vi "UI.vi"() -> ()   [LabVIEW 2017]
uses:
  <vilib>/vision/NI_Vision_Development_Module.lvlib
panel:
  out "Left side points":dbl[][](array[numeric])
  out "Bottom side points":dbl[][](array[numeric])
  out "Right side points":dbl[][](array[numeric])
  out "Top side points":dbl[][](array[numeric])
  out "time image processing":u32
  out "time load image":u32
  out "main Y":dbl[](array[numeric])
  out "main X":dbl[](array[numeric])
  out "corner":dbl[][](array[numeric])
  out "Y Resolution":i32
  out "X Resolution":i32
  out "testing 2":T1(plugin-control)
  out "black image":T1(plugin-control)
  out "buffer image":T1(plugin-control)
  in  "Path":path
  in  "Canny Parameters":T2={"Sigma"=1.0, "HThresh"=0.7, "LThres"=0.2, "WindowSize"=9}
  in  "Range (Threshold)":cluster{"Lower value":sgl, "Upper value":sgl}={"Lower value"=73.0, "Upper value"=255.0}
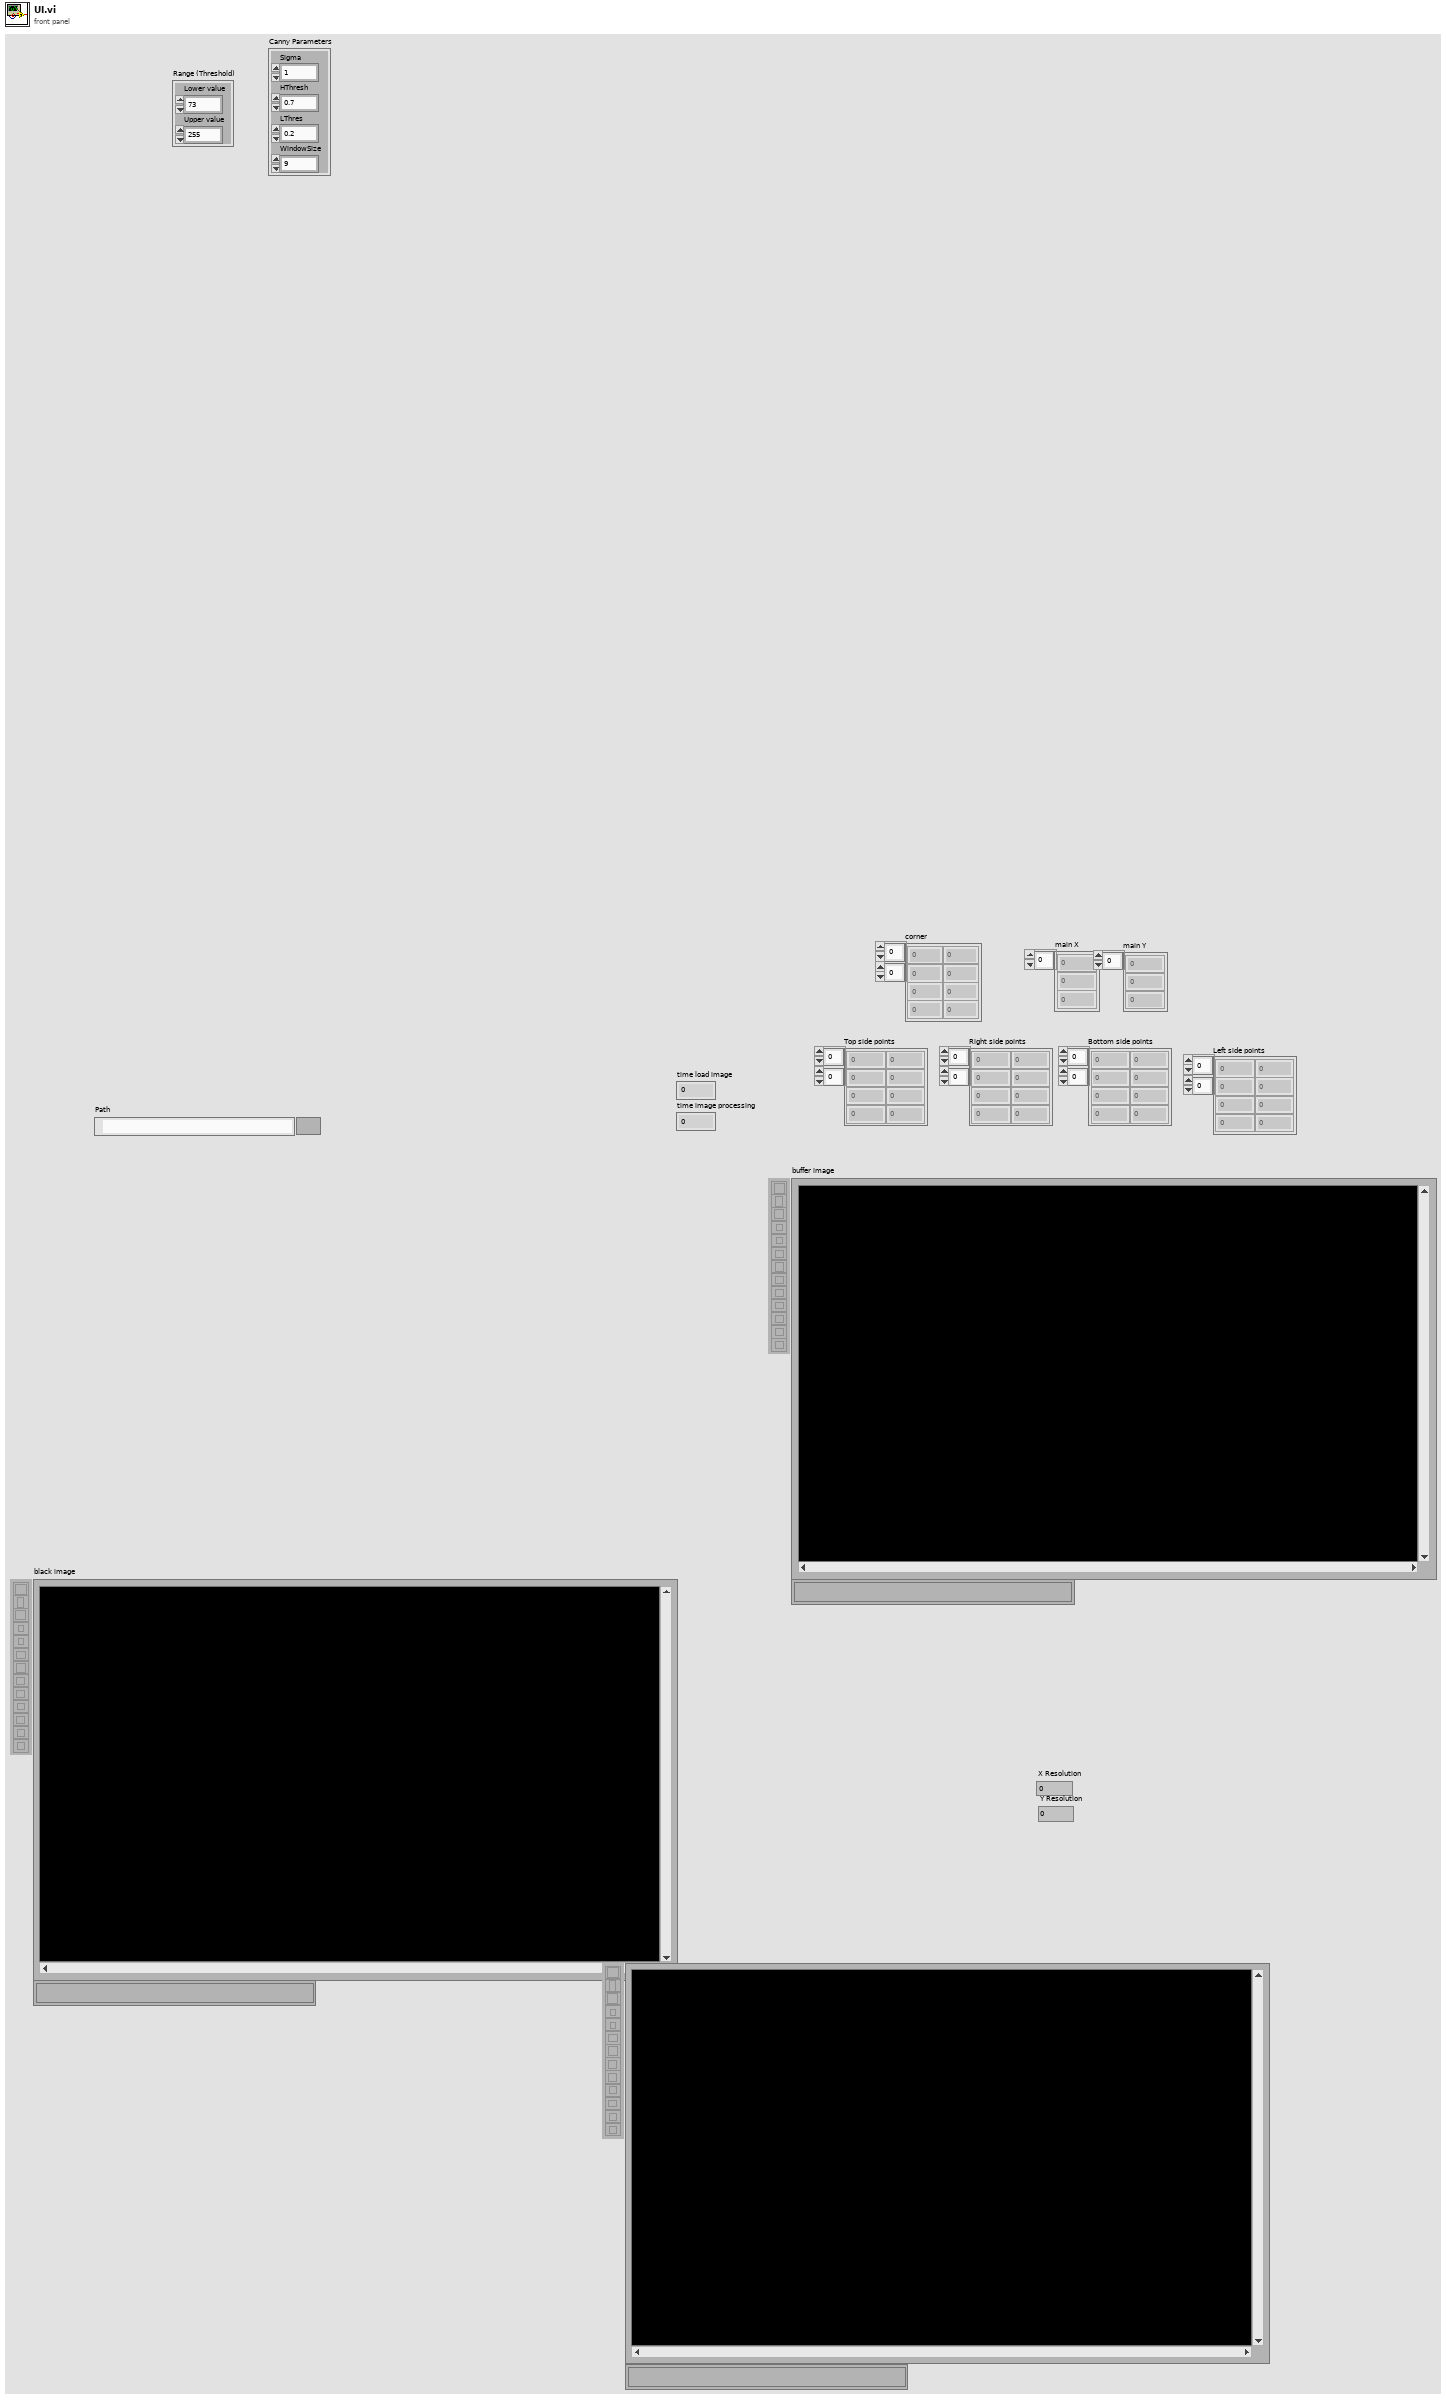
[diagram p1: front panel]
types:
  T1 = typedef "IMAQ Image.ctl" = refnum<image>
  T2 = cluster{"Sigma":sgl, "HThresh":sgl, "LThres":sgl, "WindowSize":i32}
  T3 = cluster{"Overlay?":bool, "Color":u32, "Width":u32, "Maintain Width?":bool}
  T4 = typedef "Image Type" = u32
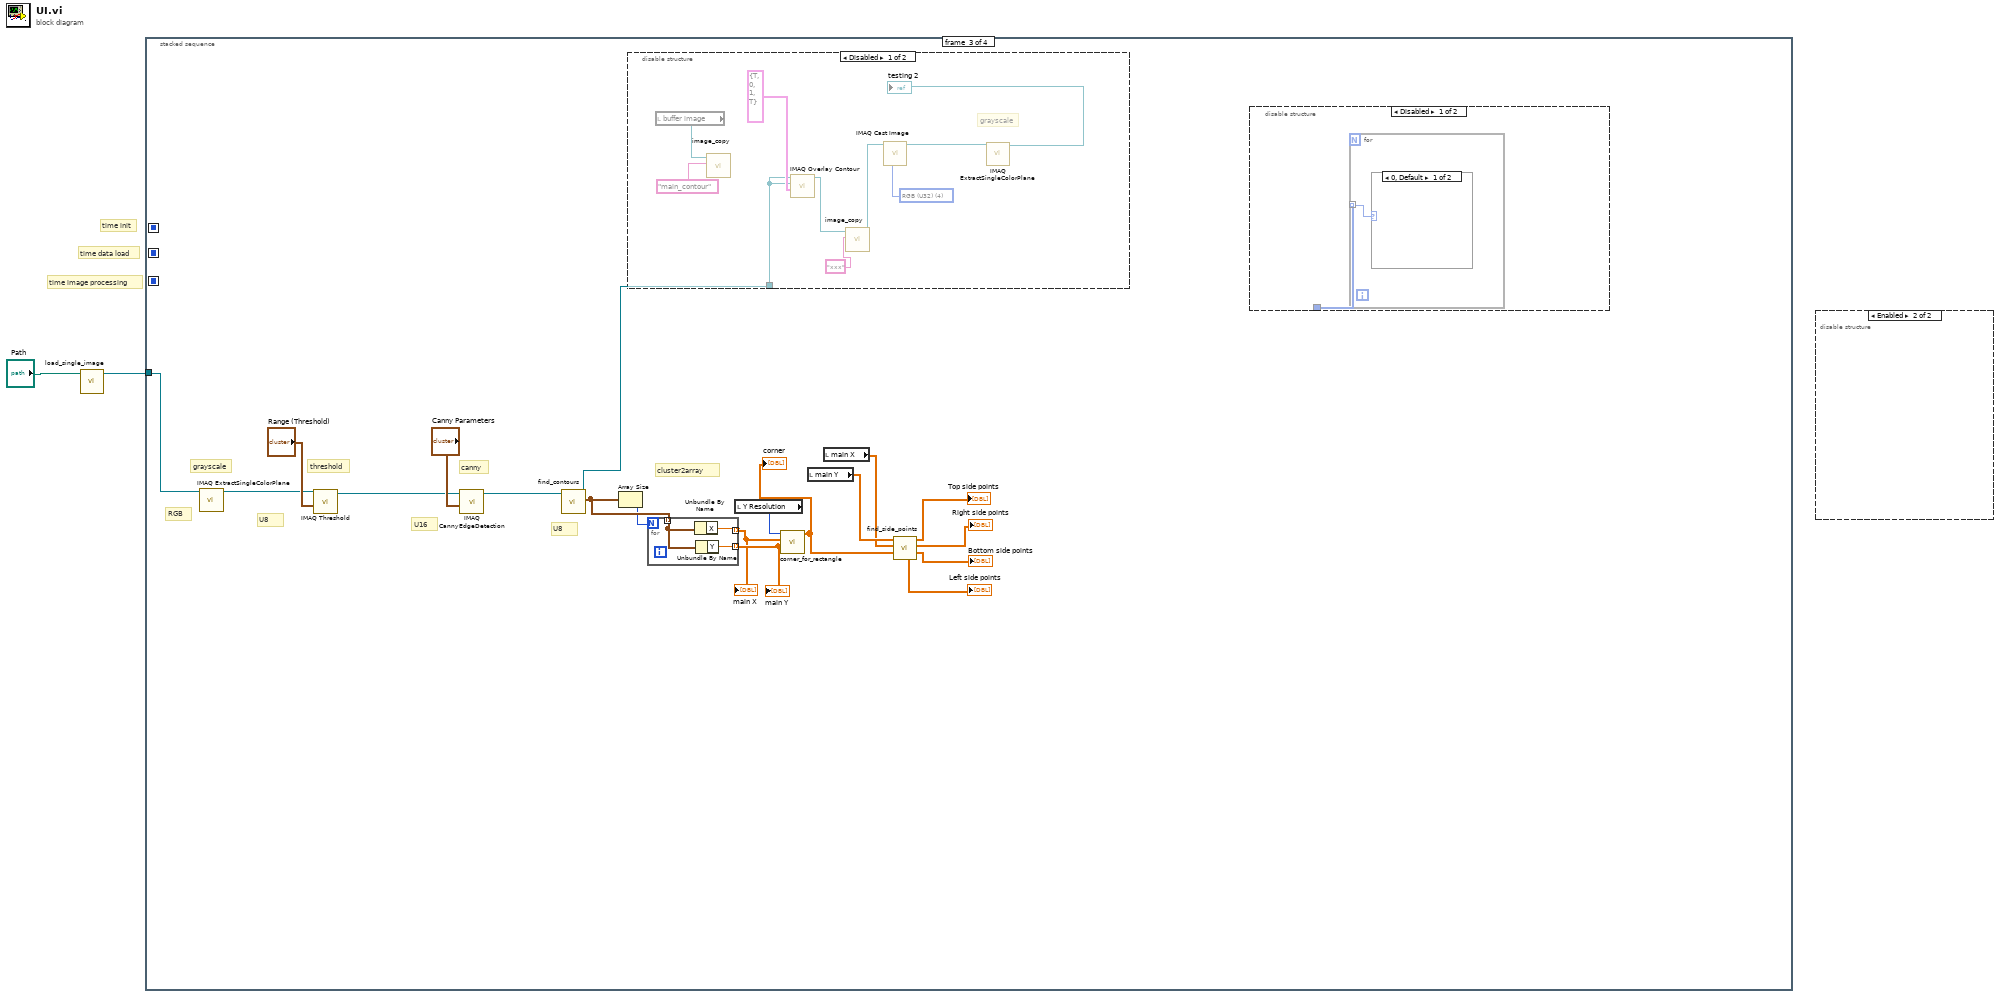
[diagram p0: block diagram]
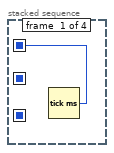
[diagram p2: hidden frame]
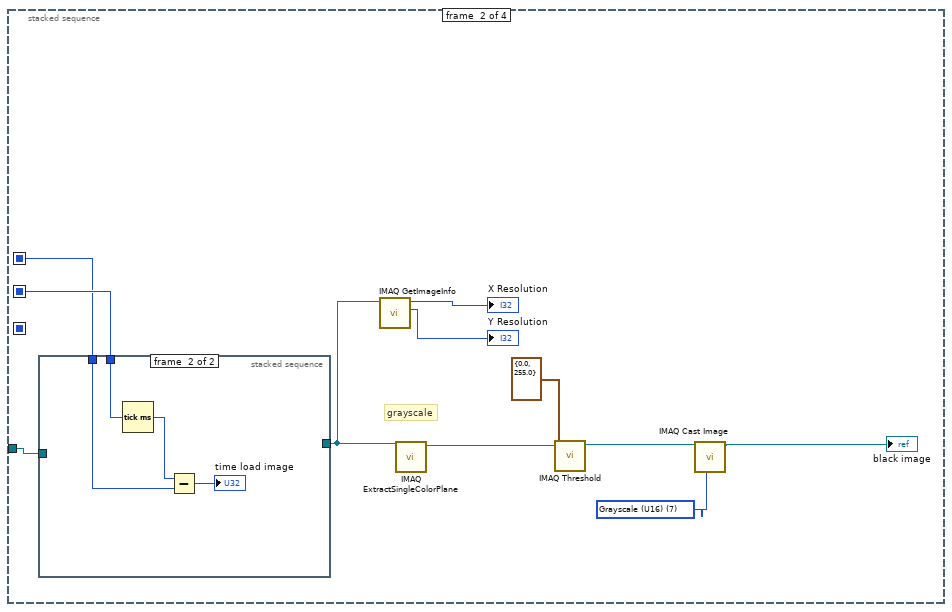
[diagram p3: hidden frame]
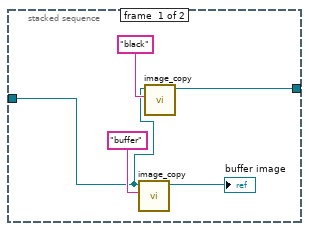
[diagram p4: hidden frame]
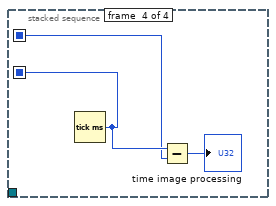
[diagram p8: hidden frame]
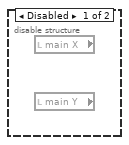
[diagram p9: hidden frame]
diagram:
  # "time image processing"
  # "time data load"
  # "time init"
  n1 = call "load_single_image.vi"("Path"="Path") -> ("Refnum out"=w1:T1)  [unwired: 10 in]
  n2 = stacked-sequence {
    seq-local: [w3 _ _ _] -> [_ w4 _ _]
    seq-local: [_ w5 _ _] -> [_ _ _ w58]
    seq-local: [_ _ _ w59] -> [_ _ _ _]
    tunnel: w1 -> [_ w6 w36 _]
    frame #0 {
      n3 = Tick Count (ms)() -> (millisecond timer value=w3:u32)
    }
    frame #1 {
      w11 = T4 7 items=["Grayscale (U8)", "Grayscale (I16)", "Grayscale (SGL)", "Complex (CSG)", "RGB (U32)", "HSL (U32)", "RGB (U64)", "Grayscale (U16)"] ("Image Type")
      # "grayscale"
      n4 = stacked-sequence {
        tunnel: [w16 _] -> w9
        tunnel: w6 -> [w15 _]
        tunnel: [_ w22] -> w5
        tunnel: w4 -> [_ w21]
        frame #0 {
          n5 = call "image_copy.vi"("buffer name"="buffer" ("Image Name"), "image in"=w15) -> ("imgae out"=→"buffer image":T1)  [unwired: 9 in]
          n6 = call "image_copy.vi"("buffer name"="black" ("Image Name"), "image in"=w15) -> ("imgae out"=w16:T1)  [unwired: 9 in]
        }
        frame #1 {
          n7 = Tick Count (ms)() -> (millisecond timer value=w22:u32)
          n8 = Subtract(x=w22, y=w21) -> (x-y=→"time load image":u32)
        }
      }
      n9 = call "IMAQ GetImageInfo"("Image"=w9) -> ("Y Resolution"=→"Y Resolution":i32, "X Resolution"=→"X Resolution":i32)  [unwired: 3 in, 6 out]
      n10 = call "IMAQ ExtractSingleColorPlane"("Image Src"=w9) -> ("Image Dst Out"=w14:T1)  [unwired: 3 in, 7 out]
      n11 = call "IMAQ Threshold"("Range"=cluster{"Lower value":sgl, "Upper value":sgl} {"Lower value"=0.0, "Upper value"=255.0}, "Image Src"=w14) -> ("Image Dst Out"=w13:T1)  [unwired: 4 in, 5 out]
      n12 = call "IMAQ Cast Image"("Image Type"=w11, "Image Src"=w13) -> ("Image Dst Out"=→"black image":T1)  [unwired: 8 in, 1 out]
    }
    frame #2 {
      # "U8"
      # "U16"
      # "U8"
      # "RGB"
      # "cluster2array"
      # "canny"
      # "threshold"
      # "grayscale"
      n13 = call "IMAQ ExtractSingleColorPlane"("Image Src"=w36) -> ("Image Dst Out"=w37:T1)  [unwired: 3 in, 7 out]
      n14 = call "IMAQ Threshold"("Range"="Range (Threshold)", "Image Src"=w37) -> ("Image Dst Out"=w39:T1)  [unwired: 4 in, 5 out]
      n15 = call "IMAQ CannyEdgeDetection"("Image Src"=w39, "Filter Parameters"="Canny Parameters") -> ("Image Dst Out"=w41:T1)  [unwired: 2 in, 5 out]
      n16 = call "find_contours.vi"("image in"=w41) -> ("Source Image Points"=w35:cluster{"X":dbl, "Y":dbl}[], "image out"=w31:T1)  [unwired: 9 in]
      n17 = Array Size(array=w35) -> (size(s)=w34:i32)
      n18 = disable-structure shown="Disabled" {
        disable-tunnel: w31 -> [w49 _]
        frame Disabled {
          w55 = T4 4 items=["Grayscale (U8)", "Grayscale (I16)", "Grayscale (SGL)", "Complex (CSG)", "RGB (U32)", "HSL (U32)", "RGB (U64)", "Grayscale (U16)"] ("Image Type")
          # "grayscale"
          n19 = local read "buffer image"() -> (w48:T1)
          n20 = call "image_copy.vi"("buffer name"="main_contour" ("Image Name"), "image in"=w48) -> ()  [unwired: 9 in, 1 out]
          n21 = call "IMAQ Overlay Contour"("Contour Points Settings"=T3 {"Overlay?"=TRUE, "Color"=0, "Width"=1, "Maintain Width?"=TRUE}, "Contour Image"=w49, "Image"=w49) -> ("Image Out"=w52:T1)  [unwired: 3 in, 5 out]
          n22 = call "image_copy.vi"("buffer name"="xxx" ("Image Name"), "image in"=w52) -> ("imgae out"=w51:T1)  [unwired: 9 in]
          n23 = call "IMAQ Cast Image"("Image Type"=w55, "Image Src"=w51) -> ("Image Dst Out"=w54:T1)  [unwired: 8 in, 1 out]
          n24 = call "IMAQ ExtractSingleColorPlane"("Image Src"=w54) -> ("Image Dst Out"=→"testing 2":T1)  [unwired: 3 in, 7 out]
        }
        frame Enabled {
        }
      }
      n25 = for {
        N: w34 -> [_]
        tunnel: w35 -> [w45] mode=indexing
        tunnel: [w46] -> w32 mode=indexing
        tunnel: [w44] -> w33 mode=indexing
        n26 = Unbundle By Name(w45) -> ("X"=w46:dbl)
        n27 = Unbundle By Name(w45) -> ("Y"=w44:dbl)
      }
      "main X" <- w32
      "main Y" <- w33
      n28 = local read "Y Resolution"() -> (w30:i32)
      n29 = call "corner_for_rectangle.vi"("Y"=w33, "X"=w32, "Y Resolution"=w30) -> ("corner"=w29:dbl[][])  [unwired: 8 in]
      "corner" <- w29
      n30 = local read "main Y"() -> (w28:dbl[])
      n31 = local read "main X"() -> (w27:dbl[])
      n32 = call "find_side_points.vi"("corner"=w29, "X  coords array"=w27, "Y coords array"=w28) -> ("Bottom side points"=→"Bottom side points":dbl[][], "Right side points"=→"Right side points":dbl[][], "Top side points"=→"Top side points":dbl[][], "Left side points"=→"Left side points":dbl[][])  [unwired: 5 in]
      n33 = disable-structure shown="Disabled" {
        disable-tunnel: _ -> [w42 _]
        frame Disabled {
          n34 = for {
            tunnel: w42 -> [w43] mode=indexing
            n35 = case shown="0, Default" w43 {
              frame 0, Default {
              }
              frame 1 {
              }
            }
          }
        }
        frame Enabled {
        }
      }
    }
    frame #3 {
      n36 = Tick Count (ms)() -> (millisecond timer value=w59:u32)
      n37 = Subtract(x=w59, y=w58) -> (x-y=→"time image processing":u32)
    }
  }
  n38 = disable-structure shown="Enabled" {
    frame Disabled {
      n39 = local read "main X"() -> ()  [unwired: 1 out]
      n40 = local read "main Y"() -> ()  [unwired: 1 out]
    }
    frame Enabled {
    }
  }
